vi "Clear-files.vi"(8 "error in (no error)":errorcluster, 11 "Object ref in":T1) -> (0 "error out":errorcluster, 3 "Object ref out":T1)   [LabVIEW 2013, in "SLMControl.lvlib" / "SC-Main.lvclass"]
uses:
  SC-Main.lvclass
  Object-reference.ctl
  UI/Control-names.ctl
  Application-status.ctl
  SC-Main.lvclass/SC-Main.ctl
  Read UI.vi
  UI/Set-control-boolean.vi
  UI/Set-control-enable-single.vi
  UI/SC-UI.lvclass
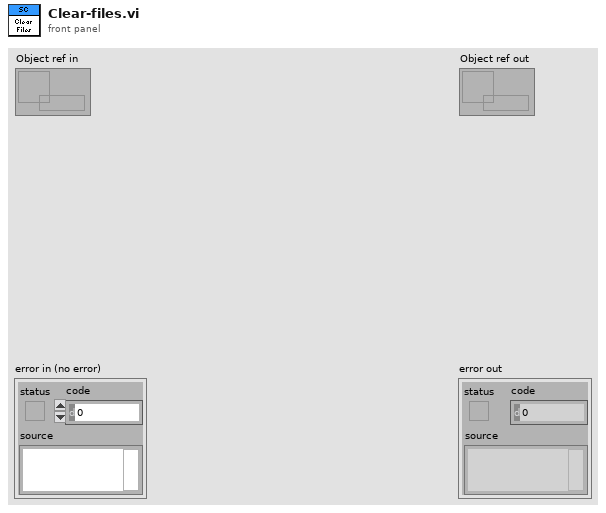
[diagram p1: front panel]
types:
  T1 = typedef "SLMControl.lvlib/SC-Main.lvclass/Object-reference.ctl" = refnum<data-value>
  T2 = typedef "SLMControl.lvlib/SC-UI.lvclass/Control-names.ctl" = enum16{"Com-in", "Com-out", "Help", "Status", "Load configuration", "Save configuration", "Load lasing files", "Load deposition files", "Clear", "Files", "Activate", "Execute", "Abort", "Options", "Current layer", "Current iteration", "Last elapsed time", "Deposition status", "Lasing job", "Status LEDs", "Exiting led", "Initialized led", "Files loaded led", "Activated led", "Executing led", "Deposition led", "Lasing job led", "Lasing led"}
  T3 = typedef "SLMControl.lvlib/SC-Main.lvclass/Application-status.ctl" = enum16{"Idle", "Initialized", "Configured", "Activated", "Started", "Paused", "Stopped", "Reset", "Error", "Exited"}
  T4 = typedef "SLMControl.lvlib/SC-UI.lvclass/Panes-reference.ctl" = refnum<data-value>
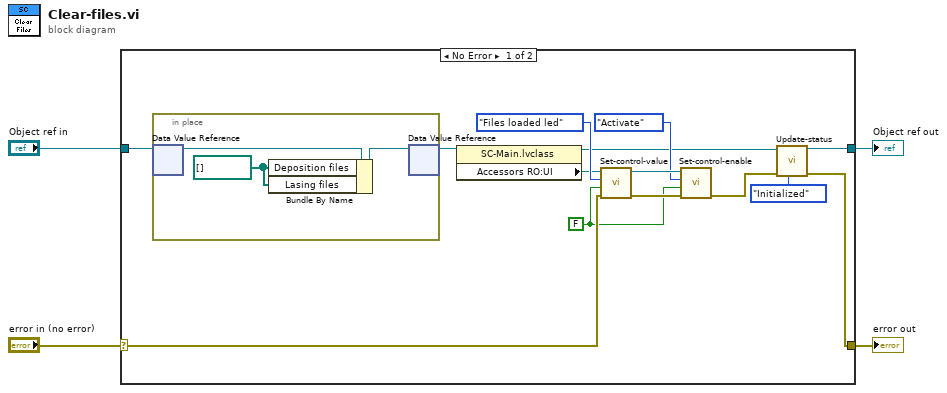
[diagram p0: block diagram]
diagram:
  n1 = case shown="No Error" "error in (no error)" {
    selector: "error in (no error)" -> [w12 w23]
    tunnel: [w8 w23] -> w3
    tunnel: [w11 w22] -> w1
    tunnel: "Object ref in" -> [w18 w22]
    frame No Error {
      w9 = FALSE ("Value")
      n2 = in-place {
        w19 = path[] [] ("Deposition files")
        n3 = in-place-dvr #1(w18) -> (w21:refnum<class "SC-Main.lvclass">)  [unwired: 1 out]
        n4 = Bundle By Name(cluster=w21, "Deposition files"=w19, "Lasing files"=w19) -> (w20:refnum<class "SC-Main.lvclass">)
        n5 = in-place-dvr #1(w20) -> (w7:T1)  [unwired: 1 out]
      }
      n6 = property class="SC-Main.lvclass"(reference=w7) -> (reference out=w5:T1, "Accessors RO:UI"=w6:T4)  [unwired: 1 in, 1 out]
      n7 = call-poly "Set-control-value.vi"("error in (no error)"=w12, "Value"=w9, "Control name"=Control-names."Files loaded led", "Panes in"=w6) -> ("error out"=w16:errorcluster, "Panes out"=w15:T4)  [unwired: 6 in]
      n8 = call-poly "Set-control-enable.vi"("error in (no error)"=w16, "Enable?"=w9, "Control name"=Control-names."Activate", "Panes in"=w15) -> ("error out"=w10:errorcluster)  [unwired: 6 in, 1 out]
      n9 = call "Update-status.vi"("Status"=Application-status."Initialized", "error in (no error)"=w10, "Object ref in"=w5) -> ("error out"=w8:errorcluster, "Object ref out"=w11:T1)  [unwired: 7 in]
    }
    frame Error {
    }
  }
  "error out" <- w3
  "Object ref out" <- w1
